vi "common msg from UAV-1.vi"() -> ()   [LabVIEW 2015, in "Biblioteka moduł map v3.lvlib" / "Zmienne.lvlib"]
uses:
  Zmienne.lvlib
panel:
  out "read messages from UAV-1":T1
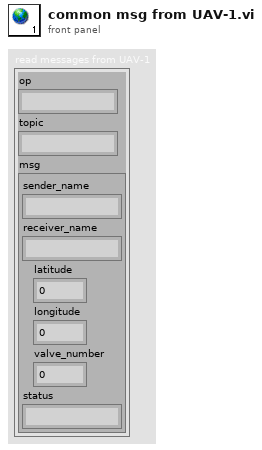
[diagram p1: front panel]
types:
  T1 = cluster{"op":string, "topic":string, "msg":cluster{"sender_name":string, "receiver_name":string, "latitude":dbl, "longitude":dbl, "valve_number":i32, "status":string}}
diagram:
